vi "Insert Queue Element anywhere in a Queue LV2012 NI Verified.vi"() -> ()   [LabVIEW 2018]
doc: "This VI inserts an item into a queue in any desired location rather than being restricted to only the begininning or the end."
panel:
  out "After new item":i32[](array[numeric])
  out "Before new item":i32[](array[numeric])
  in  "Desired Position of New Queue Item":i32 min=0 max=15
  in  "New Queue Item":i32
  # "Overview: This VI inserts an item into a queue in any desired location rather than being restricted to only the begininning or the end.\n\nRequirements: LabVIEW 2012 (or compatible).\n\nInstructions:\n1. Enter a value into New Queue Item.\n2. Select the desired position of new item.\n3. Run the VI.\n4. Check Before and After arrays."
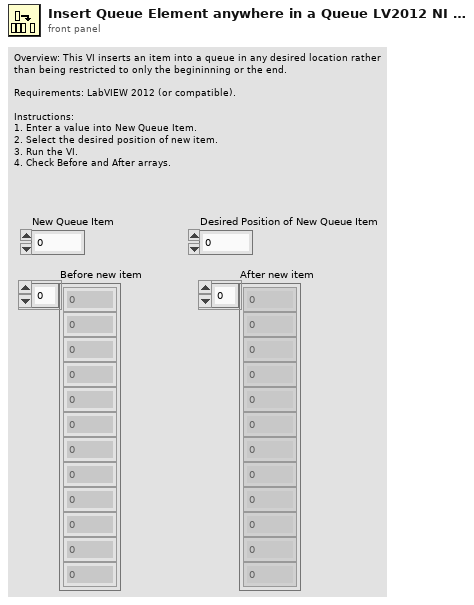
[diagram p1: front panel]
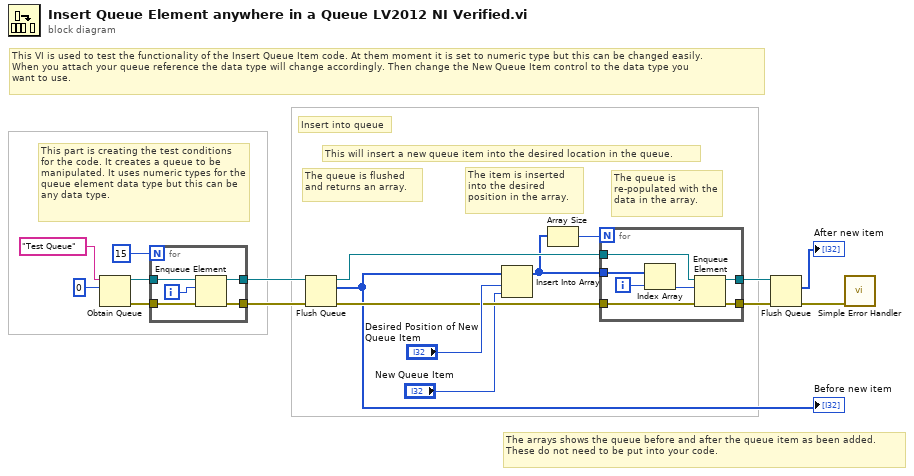
[diagram p0: block diagram]
diagram:
  # "Insert into queue"
  # "This VI is used to test the functionality of the Insert Queue Item code. At them moment it is set to numeric type but this can be changed easily. \nWhen you attach your queue reference the data type will change accordingly. Then change the New Queue Item control to the data type you\nwant to use."
  # "The arrays shows the queue before and after the queue item as been added.\nThese do not need to be put into your code."
  # "This part is creating the test conditions for the code. It creates a queue to be manipulated. It uses numeric types for the queue element data type but this can be any data type."
  # "The queue is re-populated with the data in the array."
  # "The item is inserted into the desired position in the array."
  # "The queue is flushed and returns an array."
  # "This will insert a new queue item into the desired location in the queue."
  n1 = Obtain Queue(name (unnamed)="Test Queue", element data type=0) -> (queue out=w16:refnum<queue>, error out=w5:errorcluster)  [unwired: 3 in, 1 out]
  n2 = for {
    N: 15 -> [_]
    tunnel: w16 -> [w23]
    tunnel: [w21] -> w10
    tunnel: [w20] -> w6
    tunnel: w5 -> [w19]
    i -> [w22]
    n3 = Enqueue Element(queue=w23, element=w22, error in (no error)=w19) -> (queue out=w21:refnum<queue>, error out=w20:errorcluster)  [unwired: 2 out]
  }
  n4 = Flush Queue(queue=w10, error in (no error)=w6) -> (queue out=w13:refnum<queue>, remaining elements=w1:i32[], error out=w7:errorcluster)
  "Before new item" <- w1
  n5 = Insert Into Array(array=w1, index="Desired Position of New Queue Item", new element="New Queue Item") -> (w12:i32[])
  n6 = Array Size(array=w12) -> (size(s)=w11:i32)
  n7 = for {
    N: w11 -> [_]
    tunnel: w12 -> [w30]
    tunnel: w13 -> [w27]
    tunnel: [w26] -> w9
    tunnel: [w25] -> w8
    tunnel: w7 -> [w24]
    i -> [w29]
    n8 = Index Array(array=w30, index=w29) -> (element=w28:i32)
    n9 = Enqueue Element(queue=w27, element=w28, error in (no error)=w24) -> (queue out=w26:refnum<queue>, error out=w25:errorcluster)  [unwired: 2 out]
  }
  n10 = Flush Queue(queue=w9, error in (no error)=w8) -> (remaining elements=→"After new item":i32[], error out=w4:errorcluster)  [unwired: 1 out]
  n11 = call <vilib>:"Simple Error Handler.vi"("error in (no error)"=w4) -> ()  [unwired: 1 in, 8 out]
